vi "manual_AutoDetectModules.vi"() -> ()   [LabVIEW 2017]
uses:
  Type Defs/Host - HW Config.ctl
  Type Defs/Host - Local Chassis.ctl
  Type Defs/Host - Module.ctl
  Type Defs/Host - Master.ctl
  Type Defs/Host - Slave.ctl
  Type Defs/ECAT Channel Data Type.ctl
  Scan Engine Custom Device.lvlib
  <resource>/objmgr/ni.var.rc
panel:
  out "Array":T1[](array[typedef])
  out "HW Config":T2
  in  "IP address":string="10.96.1.144s"
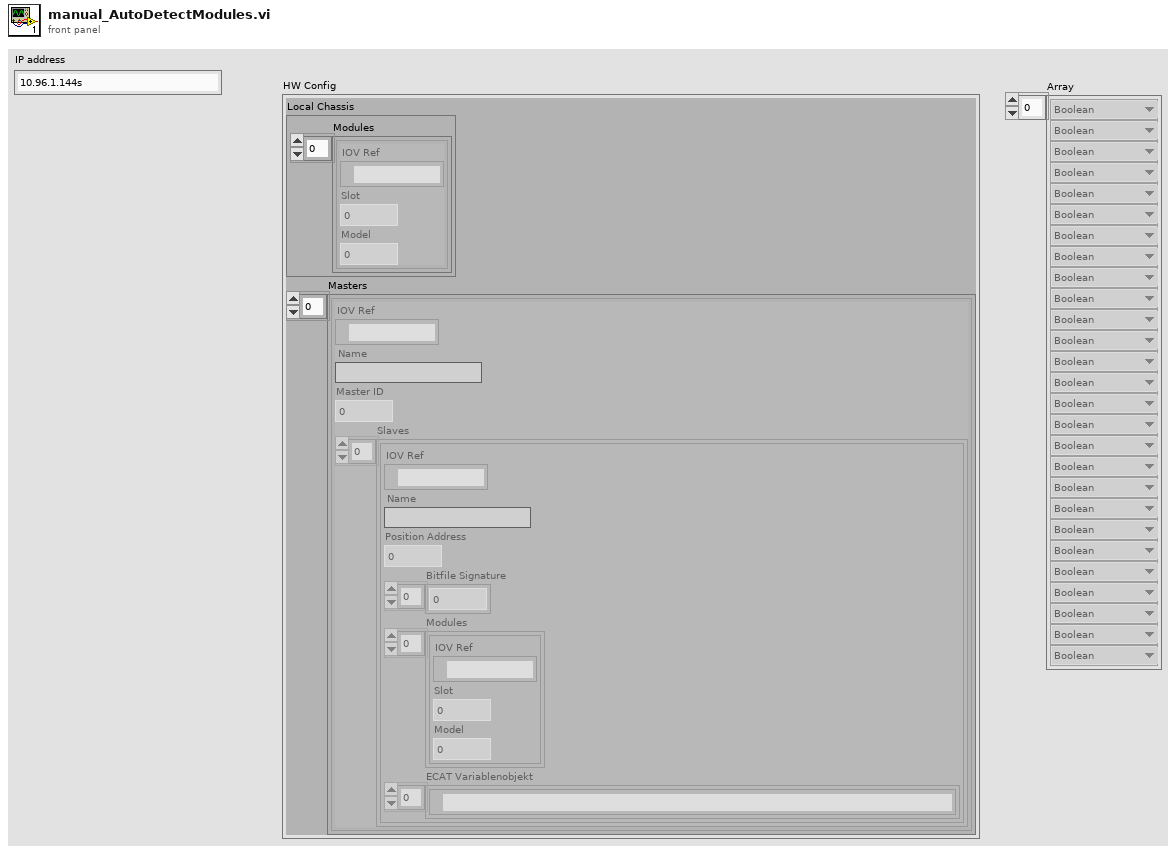
[diagram p1: front panel]
types:
  T1 = typedef "Scan Engine Custom Device.lvlib/ECAT Channel Data Type.ctl" = enum16{"Boolean", "Fixed Point", "Int8", "Int16", "Int32", "Int64", "U32 Bit Field", "UInt8", "UInt16", "UInt32", "UInt64", "Other", "DBL", "SGL"}
  T2 = typedef "Scan Engine Custom Device.lvlib/Host - HW Config.ctl" = cluster{"Local Chassis":T3, "Masters":T5[]}
  T3 = typedef "Scan Engine Custom Device.lvlib/Host - Local Chassis.ctl" = cluster{"Modules":T4[]}
  T4 = typedef "Scan Engine Custom Device.lvlib/Host - Module.ctl" = cluster{"IOV Ref":refnum<k21>, "Slot":u32, "Model":u32}
  T5 = typedef "Scan Engine Custom Device.lvlib/Host - Master.ctl" = cluster{"IOV Ref":refnum<k21>, "Name":string, "Master ID":u32, "Slaves":T6[]}
  T6 = typedef "Scan Engine Custom Device.lvlib/Host - Slave.ctl" = cluster{"IOV Ref":refnum<k21>, "Name":string, "Position Address":u16, "Bitfile Signature":u8[], "Modules":T4[], "ECAT Variablenobjekt":refnum<k21>[]}
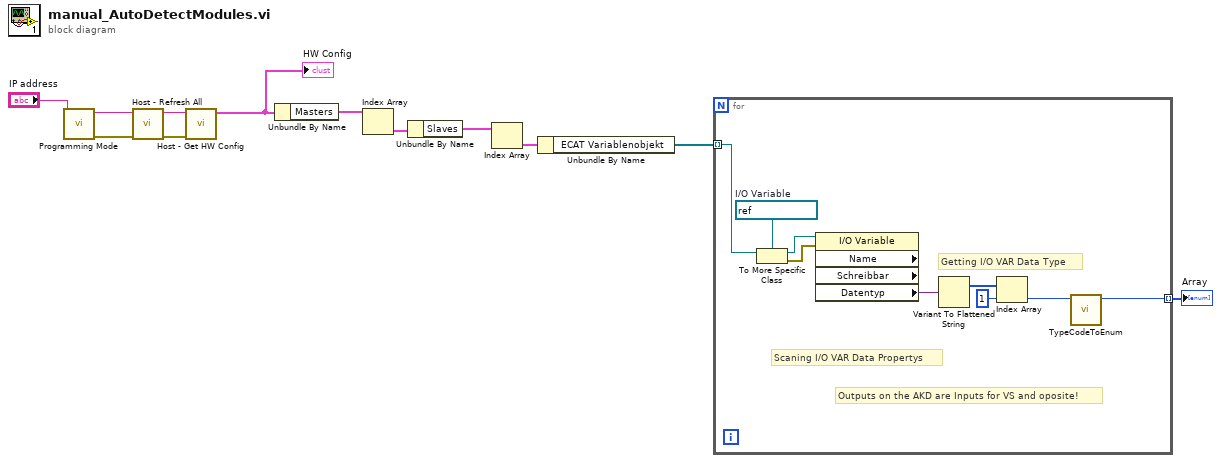
[diagram p0: block diagram]
diagram:
  n1 = call "Programming Mode.vi"("serverName In"="IP address") -> ("error out"=w12:errorcluster, "serverName Out"=w11:string)  [unwired: 9 in]
  n2 = call "Host - Refresh All.vi"("error in (no error)"=w12, "serverName"=w11) -> ("error out"=w9:errorcluster, "serverName"=w10:string)  [unwired: 8 in]
  n3 = call "Host - Get HW Config.vi"("error in (no error)"=w9, "serverName"=w10) -> ("HW Config"=w7:T2)  [unwired: 8 in, 1 out]
  "HW Config" <- w7
  n4 = Unbundle By Name(w7) -> ("Masters"=w6:T5[])
  n5 = Index Array(array=w6) -> (element=w5:T5)  [unwired: 1 in]
  n6 = Unbundle By Name(w5) -> ("Slaves"=w4:T6[])
  n7 = Index Array(array=w4) -> (element=w3:T6)  [unwired: 1 in]
  n8 = Unbundle By Name(w3) -> ("ECAT Variablenobjekt"=w2:refnum<k21>[])
  n9 = for {
    tunnel: w2 -> [w21] mode=indexing
    tunnel: [w13] -> w1 mode=indexing
    w20 = refnum<k21> refnum  # I/O Variable
    # "Getting I/O VAR Data Type"
    # "Scaning I/O VAR Data Propertys"
    # "Outputs on the AKD are Inputs for VS and oposite!"
    n10 = To More Specific Class(target class=w20, reference=w21) -> (specific class reference=w19:refnum<k21>, error out=w18:errorcluster)  [unwired: 1 in]
    n11 = property class="I/O Variable" props=["Name", "Schreibbar", "Datentyp"](reference=w19, error in=w18) -> ("Datentyp"=w17:variant)  [unwired: 4 out]
    n12 = Variant To Flattened String(Variant=w17) -> (1:w16:i16[])  [unwired: 1 out]
    n13 = Index Array(array=w16, index=1) -> (element=w14:i16)
    n14 = call "TypeCodeToEnum.vi"("Type Code (numbers in hexadecimal)"=w14) -> ("UDV Data Type"=w13:T1)  [unwired: 9 in, 1 out]
  }
  "Array" <- w1
